vi "Read (Single Point).vi"(8 "error in (no error)":errorcluster, 11 "VISA resource name":refnum<visa-resource-name>) -> (0 "error out":errorcluster, 2 "Measurement":dbl, 3 "VISA resource name out":refnum<visa-resource-name>)   [LabVIEW 2014, in "Fluke 884X Series.lvlib"]
doc: "Reads and returns a single measurement from the instrument."
uses:
  Fluke 884X Series.lvlib
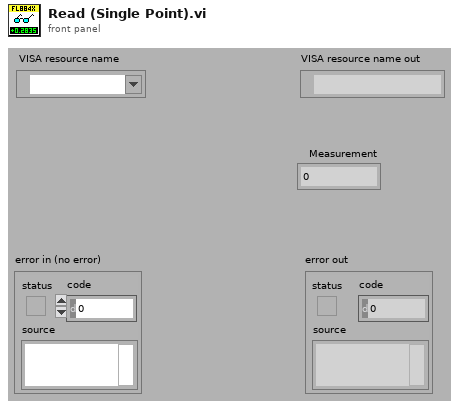
[diagram p1: front panel]
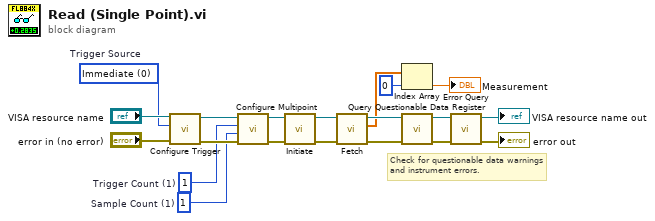
[diagram p0: block diagram]
diagram:
  w4 = 1  # Sample Count (1)
  w5 = 1  # Trigger Count (1)
  w6 = u16 0 items=["Immediate", "Software (Bus)", "External"]  # Trigger Source
  # "Check for questionable data warnings and instrument errors."
  n1 = call "Configure Trigger.vi"("error in (no error)"="error in (no error)", "Trigger Source (0: Immediate)"=w6, "VISA resource name"="VISA resource name") -> ("error out"=w7:errorcluster, "VISA resource name out"=w8:refnum<visa-resource-name>)  [unwired: 7 in]
  n2 = call "Configure Multipoint.vi"("error in (no error)"=w7, "Sample Count (1)"=w4, "Trigger Count (1)"=w5, "VISA resource name"=w8) -> ("error out"=w11:errorcluster, "VISA resource name out"=w10:refnum<visa-resource-name>)  [unwired: 6 in]
  n3 = call "Initiate.vi"("error in (no error)"=w11, "VISA resource name"=w10) -> ("error out"=w16:errorcluster, "VISA resource name out"=w15:refnum<visa-resource-name>)  [unwired: 8 in]
  n4 = call "Fetch.vi"("error in (no error)"=w16, "VISA resource name"=w15) -> ("error out"=w13:errorcluster, "Measurements"=w1:dbl[], "VISA resource name out"=w14:refnum<visa-resource-name>)  [unwired: 7 in]
  n5 = Index Array(array=w1, index=0) -> (element=→"Measurement":dbl)
  n6 = call "Query Questionable Data Register.vi"("error in (no error)"=w13, "VISA resource name"=w14) -> ("error out"=w17:errorcluster, "VISA resource name out"=w18:refnum<visa-resource-name>)  [unwired: 7 in, 1 out]
  n7 = call "Error Query.vi"("error in (no error)"=w17, "VISA resource name"=w18) -> ("error out"=→"error out":errorcluster, "VISA resource name out"=→"VISA resource name out":refnum<visa-resource-name>)  [unwired: 6 in, 2 out]
